vi "Directional Speed Sensor.vi"(6 "load data":T5={"max address"=0.0, "Memory"="Digital Pattern Gen Memory 0"}, 7 "settings.<user name>":T4, 8 "register bus":T2={"Speed"="Speed", "Crank Angle"="Crank Angle", "Cycle Angle"="Cycle Angle", "Crank Count"="Crank Count", "Cycle Count"="Cycle Count", "1.25 MHz Counter"="1.25 MHz Counter", "Crank Rollover"="Crank Rollover", "Cycle Rollover"="Cycle Rollover", "shared settings"={"start"=0.0, "stuck limit"=0.0}} {"shared settings"."start" format="%#.15g"}, 11 "input.<user name>":T1) -> (2 "digial output":bool)   [LabVIEW 2013, in "Engine Simulation Toolkit.lvlib" / "Directional Speed.lvlib"]
doc: "Outputs a digital pulse depending on engine position and a memory holding tooth center positions. When the simulated engine position passes a tooth center position, the digital pulse stays inactive for a dwell time, and then goes active for a time depending on if the engine rotated forwards or reverse. <b> This VI should be in an SCTL</b>\n\n<b>settings.<user name></b> - settings for the component. NI VeriStand will set these values. create a control for this input. Replace <user name> with the name you wish this component to display as inside NI VeriStand. Make this name consistent for all controls, indicators, for all VIs of this component.\n<b>input.<user name></b> - input for the component. NI VeriStand will set these values. create a control for this input. Replace <user name> with the name you wish this component to display as inside NI VeriStand. Make this name consistent for all controls, indicators, for all VIs of this component.\n<b>register bus</b> - connect this input to the output of the initialize APU VI. This contains references to APU state variables like position and speed.\n<b>load data</b> - This data comes from Load Directional Speed Sensor.vi\n\n<b>digital output</b> - Wire this to the digital output IO node"
uses:
  Directional Speed.lvlib
  Load Data.ctl
  Settings.ctl
  APU/Register Bus.ctl
  APU/Shared Settings.ctl
  Input.ctl
  State.ctl
  <vilib>/rvi/DataTransferAndStorage/Container/Common/niFpgaContainerExecOnDevCompGetState.vi
  <vilib>/rvi/DataTransferAndStorage/Register/Emulation/niFpgaRegisterEmulationFpgaImpl.vi
  <instcachedir>/0/niFpgaRegisterEmulationFpgaImpl_DCF4BC0110594B98B44A971D60CEEC4D.lvgen/niFpgaRegisterEmulationFpgaImpl_DCF4BC0110594B98B44A971D60CEEC4D_006.vi
  <vilib>/rvi/DataTransferAndStorage/Container/Common/niFpgaContainerGetUniqueNameForEmu.vi
  <vilib>/rvi/Memory/Memory_Emulation/nirvimemoryFastEmulationFpgaImpl.vi
  <instcachedir>/0/nirvimemoryFastEmulationFpgaImpl_5FBAB50466BC4C939F684F8805638BFC.lvgen/nirvimemoryFastEmulationFpgaImpl_5FBAB50466BC4C939F684F8805638BFC_004.vi
  <vilib>/rvi/Memory/Memory_Emulation/niFpgaMemoryEmulationCacheClearOnFirstRun.vi
  <vilib>/rvi/Memory/Memory_Emulation/nirvimemoryEmulationManagerCache_MakeExclusive.vi
  <vilib>/rvi/Memory/Memory_Emulation/niFpgaMemoryEmulationValidateCache.vi
  <vilib>/rvi/Memory/Memory_Emulation/nirvimemoryEmulationManagerCache_ReleaseExclusive.vi
  <vilib>/rvi/Memory/Memory_Emulation/nirvimemoryEmulationManagerCache_InsertValue.vi
  <vilib>/Utility/error.llb/Clear Errors.vi
  <vilib>/rvi/Memory/Memory_Emulation/nirvimemoryEmulationManagerCache_GetValue.vi
  <vilib>/rvi/DataTransferAndStorage/Container/XNode/niFpgaContainer.xnode
  <vilib>/rvi/DataTransferAndStorage/Register/Emulation/niFpgaRegisterEmulationRefIn.vi
  <vilib>/rvi/Memory/Memory_Emulation/niFpgaMemoryEmulationRefIn.vi
  APU/APU.lvlib
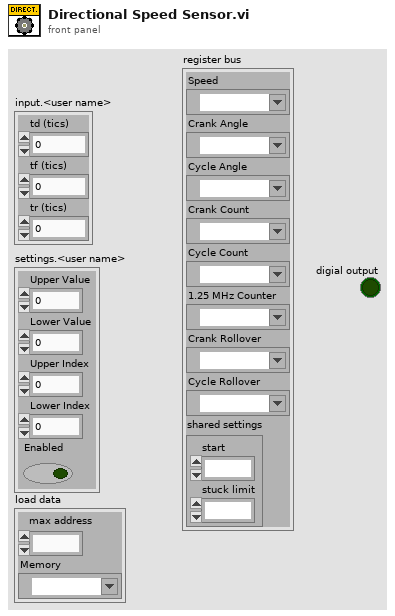
[diagram p1: front panel]
types:
  T1 = typedef "Engine Simulation Toolkit.lvlib/Directional Speed.lvlib/Input.ctl" = cluster{"td (tics)":u16, "tf (tics)":u16, "tr (tics)":u16}
  T2 = typedef "Engine Simulation Toolkit.lvlib/APU.lvlib/Register Bus.ctl" = cluster{"Speed":refnum<k21>, "Crank Angle":refnum<k21>, "Cycle Angle":refnum<k21>, "Crank Count":refnum<k21>, "Cycle Count":refnum<k21>, "1.25 MHz Counter":refnum<k21>, "Crank Rollover":refnum<k21>, "Cycle Rollover":refnum<k21>, "shared settings":T3}
  T3 = typedef "Engine Simulation Toolkit.lvlib/APU.lvlib/Shared Settings.ctl" = cluster{"start":fxp<+,17,17>, "stuck limit":fxp<+,18,18>}
  T4 = typedef "Engine Simulation Toolkit.lvlib/Directional Speed.lvlib/Settings.ctl" = cluster{"Upper Value":u16, "Lower Value":u16, "Upper Index":fxp<+,10,10>, "Lower Index":fxp<+,10,10>, "Enabled":bool}
  T5 = typedef "Engine Simulation Toolkit.lvlib/Directional Speed.lvlib/Load Data.ctl" = cluster{"max address":fxp<+,10,10>, "Memory":refnum<k21>}
  T6 = typedef "Engine Simulation Toolkit.lvlib/Directional Speed.lvlib/State Data.ctl" = cluster{"settings.<user name>":T4, "State":T7}
  T7 = typedef "Engine Simulation Toolkit.lvlib/Directional Speed.lvlib/State.ctl" = enum8{"Init", "Detect", "Positive Move td", "Negative Move td", "tf", "tr"}
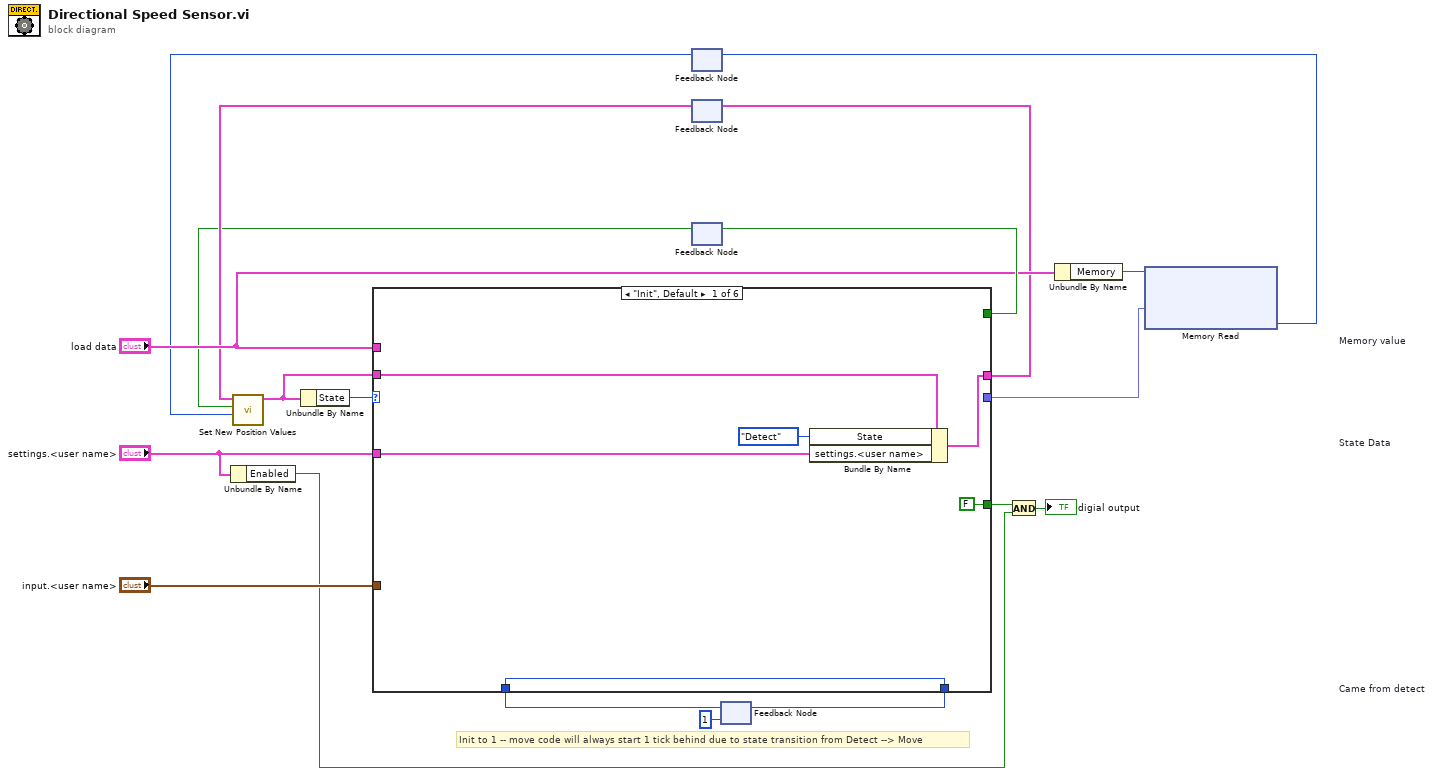
[diagram p0: block diagram]
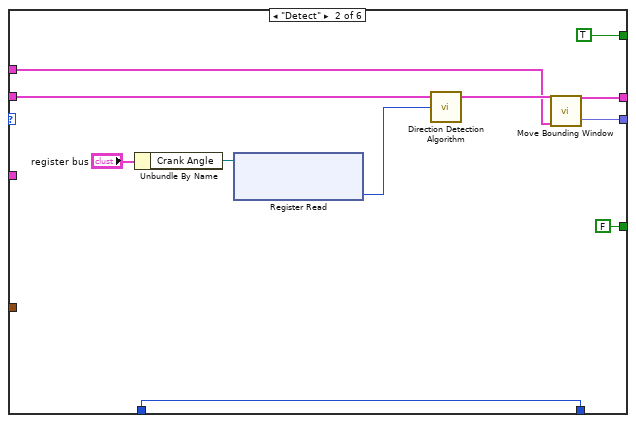
[diagram p2: hidden frame]
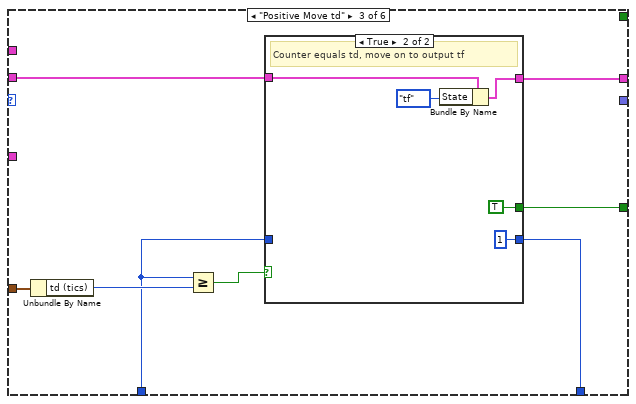
[diagram p3: hidden frame]
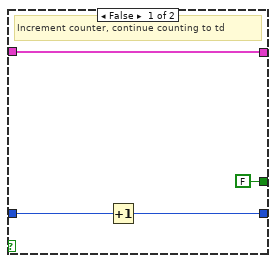
[diagram p4: hidden frame]
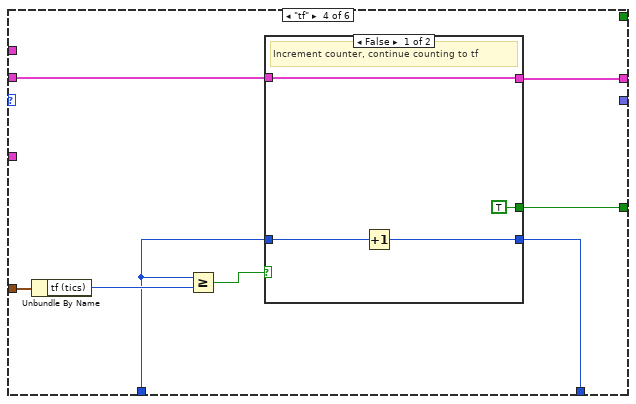
[diagram p5: hidden frame]
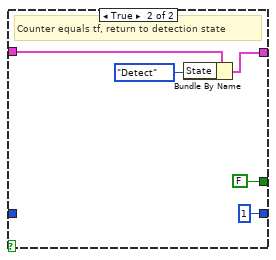
[diagram p6: hidden frame]
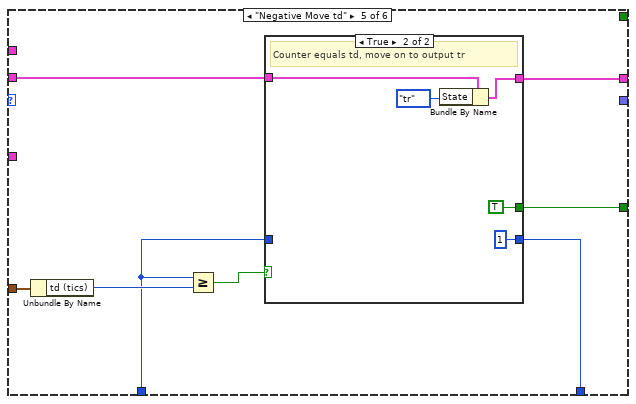
[diagram p7: hidden frame]
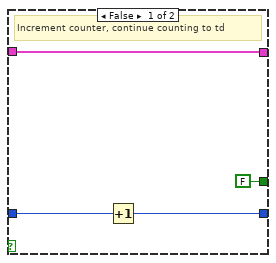
[diagram p8: hidden frame]
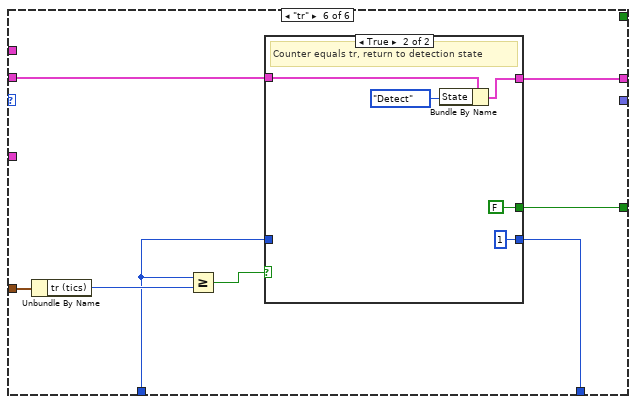
[diagram p9: hidden frame]
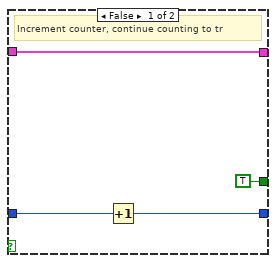
[diagram p10: hidden frame]
diagram:
  # "Init to 1 -- move code will always start 1 tick behind due to state transition from Detect --> Move"
  n1 = Unbundle By Name("settings.<user name>") -> ("Enabled"=w1:bool)
  n2 = feedback #1 "Memory value"() -> (w10:u16)  [unwired: 1 in]
  n3 = feedback #2 "State Data"() -> (w8:T6)  [unwired: 1 in]
  n4 = feedback #3 "Came from detect"() -> (w7:bool)  [unwired: 1 in]
  n5 = call "Set New Position Values.vi"("Data"=w10, "Came From Detect?"=w7, "State Data in"=w8) -> ("State Data out"=w5:T6)  [unwired: 8 in]
  n6 = Unbundle By Name(w5) -> ("State"=w9:T7)
  n7 = feedback #4(u16 1) -> (w16:u16)
  n8 = case shown="\"Init\", Default" w9 {
    tunnel: w5 -> [w25 w36 w40 w57 w74 w91]
    tunnel: [w23 w34 w39 w56 w73 w90] -> w12
    tunnel: "input.<user name>" -> [_ _ w44 w61 w78 w95]
    tunnel: [FALSE FALSE w42 w59 w76 w93] -> w18
    tunnel: [w21 w29 w37 w55 w72 w88] -> w17
    tunnel: w16 -> [w21 w29 w38 w54 w71 w89]
    tunnel: [_ TRUE _ _ _ _] -> w15
    tunnel: "load data" -> [_ w27 _ _ _ _]
    tunnel: [_ w26 _ _ _ _] -> w6
    tunnel: "settings.<user name>" -> [w20 _ _ _ _ _]
    frame "Init", Default {
      n9 = Bundle By Name(cluster=w25, "State"=State."Detect", "settings.<user name>"=w20) -> (w23:T6)
    }
    frame "Detect" {
      n10 = Unbundle By Name("register bus") -> ("Crank Angle"=w32:refnum<k21>)
      n11 = xnode ("Register Read")("Register In"=w32) -> ("Data"=w31:u16)  [unwired: 1 out]
      n12 = call "Direction Detection Algorithm.vi"("Current Position"=w31, "State Data in"=w36) -> ("State Data Out"=w35:T6)  [unwired: 3 in]
      n13 = call "Move Bounding Window.vi"("load data"=w27, "State Data"=w35) -> ("Memory Lookup"=w26:fxp<+,10,10>, "State Data Out"=w34:T6)  [unwired: 2 in]
    }
    frame "Positive Move td" {
      n14 = Unbundle By Name(w44) -> ("td (tics)"=w41:u16)
      n15 = Greater Or Equal?(x=w38, y=w41) -> (x >= y?=w43:bool)
      n16 = case shown="True" w43 {
        tunnel: [FALSE TRUE] -> w42
        tunnel: w38 -> [w48 _]
        tunnel: [w47 u16 1] -> w37
        tunnel: w40 -> [w45 w50]
        tunnel: [w45 w49] -> w39
        frame False {
          # "Increment counter, continue counting to td"
          n17 = Increment(x=w48) -> (x+1=w47:u16)
        }
        frame True {
          # "Counter equals td, move on to output tf"
          n18 = Bundle By Name(cluster=w50, "State"=State."tf") -> (w49:T6)
        }
      }
    }
    frame "tf" {
      n19 = Unbundle By Name(w61) -> ("tf (tics)"=w58:u16)
      n20 = Greater Or Equal?(x=w54, y=w58) -> (x >= y?=w60:bool)
      n21 = case shown="False" w60 {
        tunnel: [TRUE FALSE] -> w59
        tunnel: w54 -> [w65 _]
        tunnel: [w64 u16 1] -> w55
        tunnel: w57 -> [w62 w67]
        tunnel: [w62 w66] -> w56
        frame False {
          # "Increment counter, continue counting to tf"
          n22 = Increment(x=w65) -> (x+1=w64:u16)
        }
        frame True {
          # "Counter equals tf, return to detection state"
          n23 = Bundle By Name(cluster=w67, "State"=State."Detect") -> (w66:T6)
        }
      }
    }
    frame "Negative Move td" {
      n24 = Unbundle By Name(w78) -> ("td (tics)"=w75:u16)
      n25 = Greater Or Equal?(x=w71, y=w75) -> (x >= y?=w77:bool)
      n26 = case shown="True" w77 {
        tunnel: [FALSE TRUE] -> w76
        tunnel: w71 -> [w82 _]
        tunnel: [w81 u16 1] -> w72
        tunnel: w74 -> [w79 w84]
        tunnel: [w79 w83] -> w73
        frame False {
          # "Increment counter, continue counting to td"
          n27 = Increment(x=w82) -> (x+1=w81:u16)
        }
        frame True {
          # "Counter equals td, move on to output tr"
          n28 = Bundle By Name(cluster=w84, "State"=State."tr") -> (w83:T6)
        }
      }
    }
    frame "tr" {
      n29 = Unbundle By Name(w95) -> ("tr (tics)"=w92:u16)
      n30 = Greater Or Equal?(x=w89, y=w92) -> (x >= y?=w94:bool)
      n31 = case shown="True" w94 {
        tunnel: [TRUE FALSE] -> w93
        tunnel: w89 -> [w99 _]
        tunnel: [w98 u16 1] -> w88
        tunnel: w91 -> [w96 w101]
        tunnel: [w96 w100] -> w90
        frame False {
          # "Increment counter, continue counting to tr"
          n32 = Increment(x=w99) -> (x+1=w98:u16)
        }
        frame True {
          # "Counter equals tr, return to detection state"
          n33 = Bundle By Name(cluster=w101, "State"=State."Detect") -> (w100:T6)
        }
      }
    }
  }
  n34 = feedback-in #2(w12) -> ()
  n35 = feedback-in #3(w15) -> ()
  n36 = feedback-in #4(w17) -> ()
  n37 = And(x=w18, y=w1) -> (x .and. y?=→"digial output":bool)
  n38 = Unbundle By Name("load data") -> ("Memory"=w13:refnum<k21>)
  n39 = xnode ("Memory Read")("Address"=w6, "Memory In"=w13) -> ("Data"=w11:u16)  [unwired: 1 out]
  n40 = feedback-in #1(w11) -> ()
